vi "SUB_COM_FLUSH_TXRX.vi"(3 "VISA resource name":refnum<visa-resource-name>) -> (1 "VISA resource name out":refnum<visa-resource-name>)   [LabVIEW 2011]
uses:
  <vilib>/Instr/_visa.llb/VISA Flush IO Buffer Mask.ctl
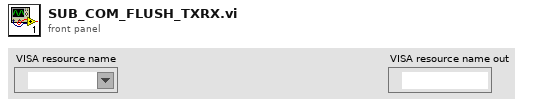
[diagram p1: front panel]
types:
  T1 = typedef "VISA Flush IO Buffer Mask.ctl" = u16
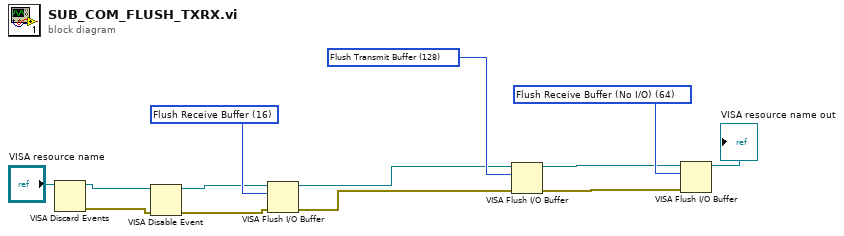
[diagram p0: block diagram]
diagram:
  w9 = T1 16 items=["Flush Receive Buffer"=16, "Write Transmit Buffer to Device"=32, "Flush Receive Buffer (No I/O)"=64, "Flush Transmit Buffer"=128] ("Mask")
  w12 = T1 64 items=["Flush Receive Buffer"=16, "Write Transmit Buffer to Device"=32, "Flush Receive Buffer (No I/O)"=64, "Flush Transmit Buffer"=128] ("Mask")
  w13 = T1 128 items=["Flush Receive Buffer"=16, "Write Transmit Buffer to Device"=32, "Flush Receive Buffer (No I/O)"=64, "Flush Transmit Buffer"=128] ("Mask")
  n1 = VISA Discard Events(11:"VISA resource name") -> (0:w3:errorcluster, 3:w7:refnum<visa-resource-name>)  [unwired: 3 in]
  n2 = VISA Disable Event(8:w3, 11:w7) -> (0:w4:errorcluster, 3:w6:refnum<visa-resource-name>)  [unwired: 2 in]
  n3 = VISA Flush I/O Buffer(VISA resource name=w6, mask (16)=w9, error in (no error)=w4) -> (VISA resource name out=w8:refnum<visa-resource-name>, error out=w5:errorcluster)
  n4 = VISA Flush I/O Buffer(VISA resource name=w8, mask (16)=w13, error in (no error)=w5) -> (VISA resource name out=w11:refnum<visa-resource-name>, error out=w10:errorcluster)
  n5 = VISA Flush I/O Buffer(VISA resource name=w11, mask (16)=w12, error in (no error)=w10) -> (VISA resource name out=→"VISA resource name out":refnum<visa-resource-name>)  [unwired: 1 out]
